vi "lamp-init.vi"(8 "error in (no error)":errorcluster, 11 "Lamp":refnum<vi>) -> (0 "error out":errorcluster, 3 "Lamp Out":refnum<vi>)   [LabVIEW 2016]
uses:
  <vilib>/Instr/_visa.llb/VISA Configure Serial Port (Instr).vi
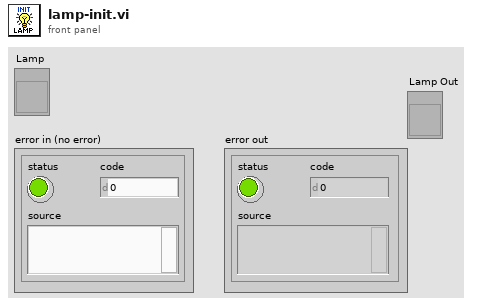
[diagram p1: front panel]
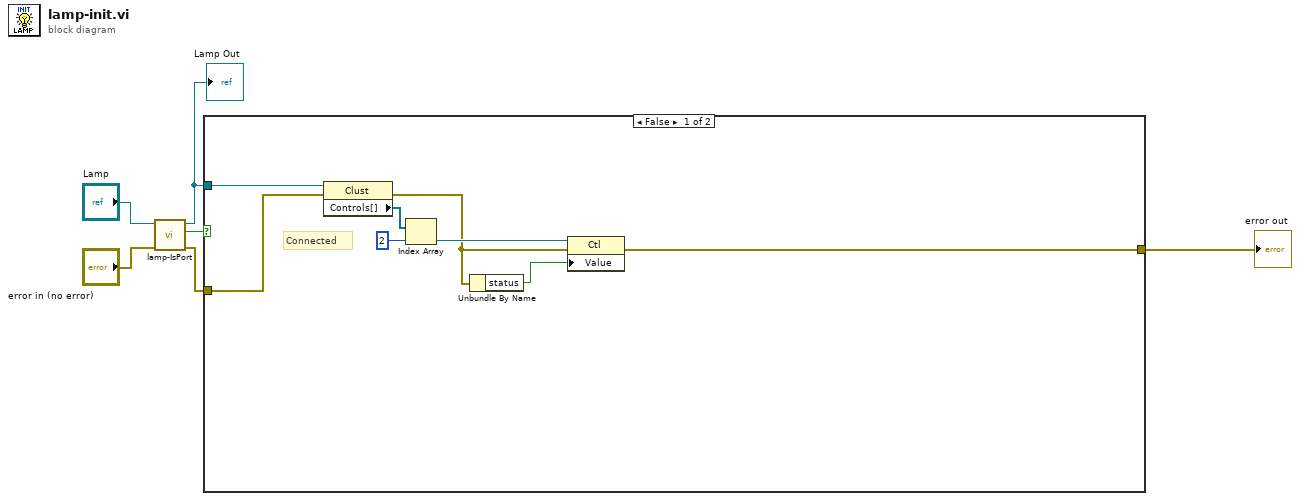
[diagram p0: block diagram]
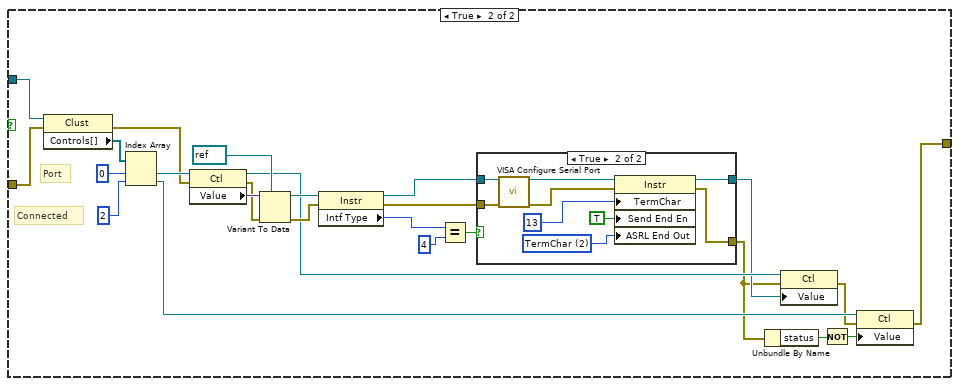
[diagram p2: hidden frame]
diagram:
  n1 = call "lamp-IsPort.vi"("error in (no error)"="error in (no error)", "Lamp"="Lamp") -> ("error out"=w4:errorcluster, "Boolean"=w3:bool, "Lamp"=w1:refnum<vi>)  [unwired: 7 in]
  "Lamp Out" <- w1
  n2 = case shown="False" w3 {
    tunnel: [w8 w15] -> w2
    tunnel: w1 -> [w12 w34]
    tunnel: w4 -> [w11 w33]
    frame False {
      # "Connected"
      n3 = property class="Clust"(reference=w12, error in=w11) -> (error out=w9:errorcluster, "Controls[]"=w14:refnum<vi>[])  [unwired: 1 out]
      n4 = Index Array(array=w14, index=2) -> (element=w10:refnum<vi>)
      n5 = Unbundle By Name(w9) -> ("status"=w7:bool)
      n6 = property class="Ctl"(reference=w10, error in=w9, "Value"=w7) -> (error out=w8:errorcluster)  [unwired: 1 out]
    }
    frame True {
      # "Connected"
      # "Port"
      n7 = property class="Clust"(reference=w34, error in=w33) -> (error out=w28:errorcluster, "Controls[]"=w32:refnum<vi>[])  [unwired: 1 out]
      n8 = Index Array(array=w32, index #1=0 ("index"), index #2=2 ("index")) -> (element #1=w29:refnum<vi>, element #2=w20:refnum<vi>)
      n9 = property class="Ctl"(reference=w29, error in=w28) -> (reference out=w22:refnum<vi>, error out=w26:errorcluster, "Value"=w27:variant)
      n10 = Variant To Data(error in=w26, type=refnum<visa-resource-name> refnum ("reference out"), Variant=w27) -> (data=w25:refnum<visa-resource-name>, error out=w24:errorcluster)
      n11 = property class="Instr"(reference=w25, error in=w24) -> (reference out=w39:refnum<visa-resource-name>, error out=w38:errorcluster, "Intf Type"=w35:u16)
      n12 = Equal?(x=w35, y=u16 4) -> (x = y?=w37:bool)
      n13 = case shown="True" w37 {
        tunnel: w38 -> [w41 w50]
        tunnel: w39 -> [w40 w49]
        tunnel: [w41 w46] -> w16
        tunnel: [w40 w42] -> w21
        frame False {
        }
        frame True {
          w43 = u16 2 items=["None", "Last Bit", "TermChar", "Break"] ("Serial Settings:End Mode for Writes")
          n14 = call-poly "VISA Configure Serial Port"("VISA resource name"=w49, "error in (no error)"=w50) -> ("VISA resource name out"=w48:refnum<visa-resource-name>, "error out"=w47:errorcluster)  [unwired: 12 in]
          n15 = property class="Instr"(reference=w48, error in=w47, "TermChar"=u8 13 ("Message Based Settings:Termination Character"), "Send End En"=TRUE ("Message Based Settings:Send End Enable"), "ASRL End Out"=w43) -> (reference out=w42:refnum<visa-resource-name>, error out=w46:errorcluster)
        }
      }
      n16 = Unbundle By Name(w16) -> ("status"=w18:bool)
      n17 = property class="Ctl"(reference=w22, error in=w16, "Value"=w21) -> (error out=w19:errorcluster)  [unwired: 1 out]
      n18 = Not(x=w18) -> (.not. x?=w17:bool)
      n19 = property class="Ctl"(reference=w20, error in=w19, "Value"=w17) -> (error out=w15:errorcluster)  [unwired: 1 out]
    }
  }
  "error out" <- w2
